vi "ucno_call objective function.vi"(5 "function and data":T2, 6 "output control":T1, 8 "error in (no error)":errorcluster, 11 "X":dbl[](array[numeric])) -> (0 "error out":errorcluster, 1 "number of function evaluations":i32, 2 "gradient":dbl[](array[numeric]), 3 "f(X)":dbl)   [LabVIEW 2017, in "NI_Gmath.lvlib"]
uses:
  NI_Gmath.lvlib
  ucno_user function ref and data.ctl
  ucno_user objective function ref.ctl
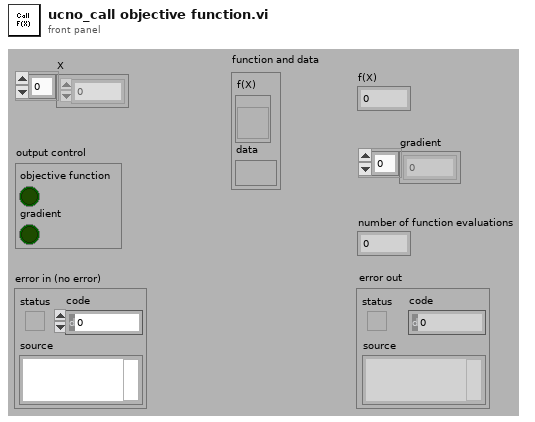
[diagram p1: front panel]
types:
  T1 = cluster{"objective function":bool, "gradient":bool}
  T2 = typedef "NI_Gmath.lvlib/ucno_user function ref and data.ctl" = cluster{"f(X)":T3, "data":variant}
  T3 = typedef "NI_Gmath.lvlib/ucno_user objective function ref.ctl" = refnum<vi>
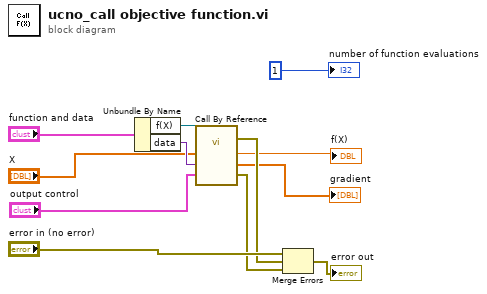
[diagram p0: block diagram]
diagram:
  n1 = Unbundle By Name("function and data") -> ("f(X)"=w7:T3, "data"=w3:variant)
  n2 = call-by-ref "?"(reference=w7, "output control"="output control", "data"=w3, "X"="X") -> (error out=w10:errorcluster, 0:"error out"=w6:errorcluster, "gradient"=→"gradient":dbl[], "f(X)"=→"f(X)":dbl)  [unwired: 1 in, 1 out]
  n3 = Merge Errors("error in (no error)", w10, w6) -> (→"error out":errorcluster)
  "number of function evaluations" <- 1
